vi "Version_Parse.vi"(0 "All_ERD_Data_Bundled_Brass in":T2, 5 "Converted Data Out":T1 {"CRC" format="%04x"; "Length" format="%02x"; "Command" format="%02x"; "Destination" format="%02x"; "Source" format="%02x"}, 11 "Error In":errorcluster) -> (4 "All_ERD_Data_Bundled_Brass out":T2, 15 "Error Out":errorcluster)   [LabVIEW 2019]
uses:
  type defs/All_Bundled_Data_JL.ctl
  type defs/Version.ctl
  type defs/ERD_Always_Show_JL.ctl
  type defs/CSV_File_String_Arrays.ctl
  type defs/Fault Table Array.ctl
  type defs/Fault_Table_Info.ctl
  type defs/Heat Control.ctl
  type defs/ERD_Commercial_Laundry.ctl
  type defs/BootloaderVersion.ctl
  type defs/ERD_RJ45.ctl
  Common/LabVIEW GEA2 Toolkit/GEA3/type defs/Data Out.ctl
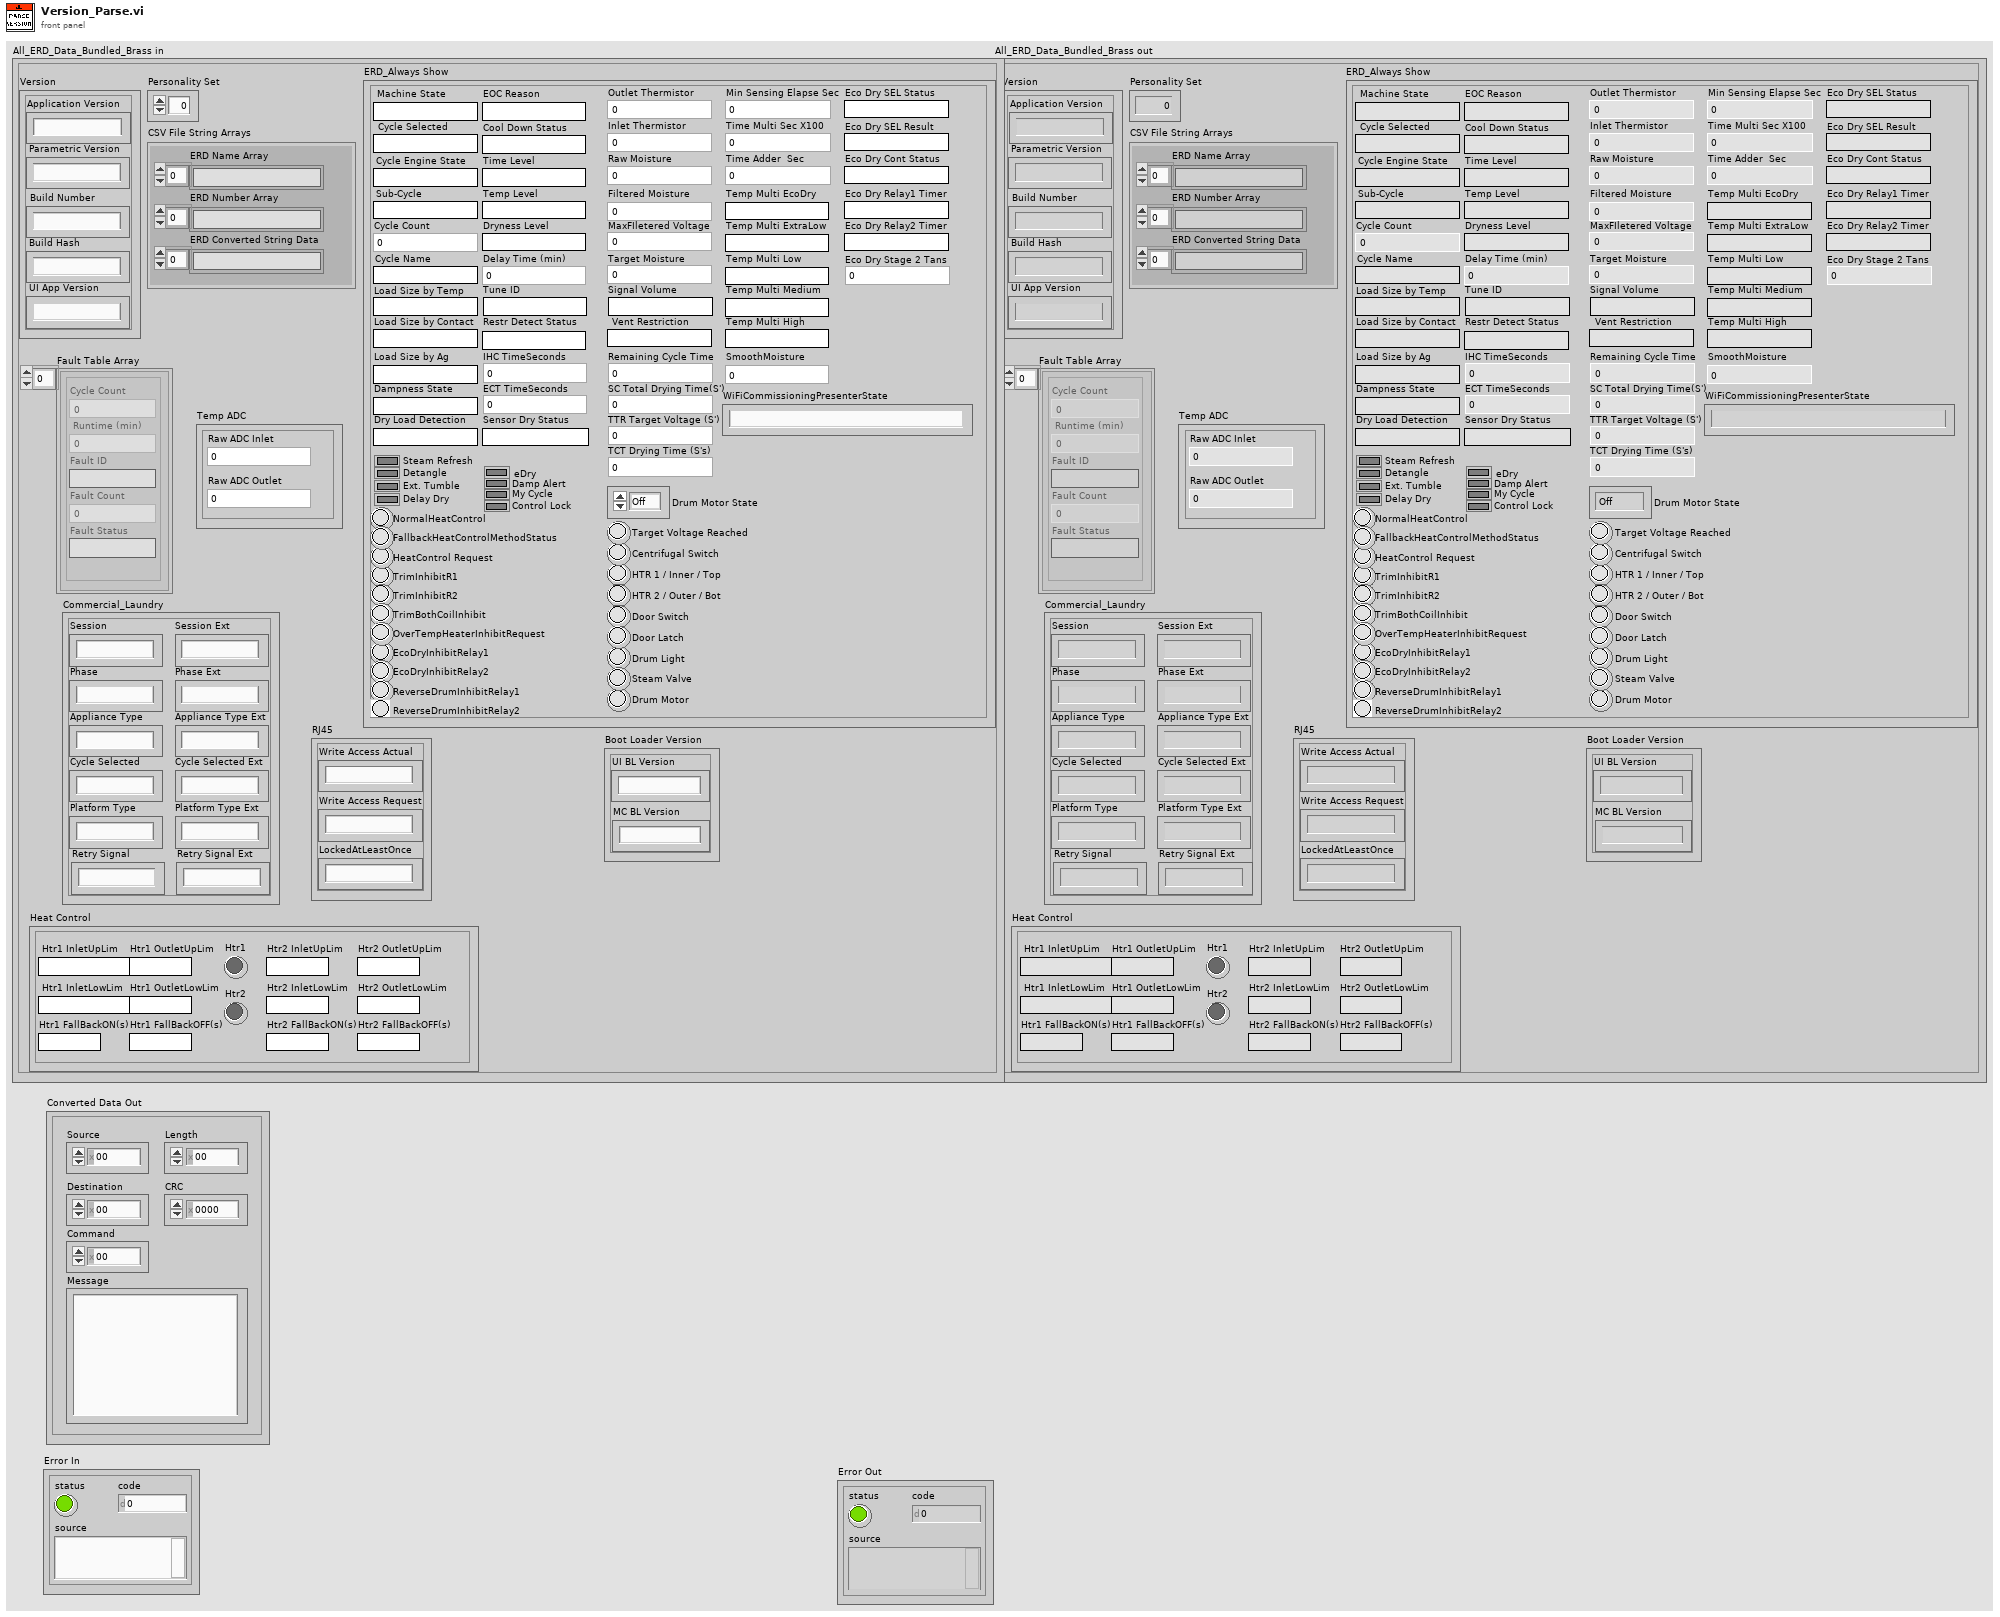
[diagram p1: front panel]
types:
  T1 = typedef "Data Out.ctl" = cluster{"Source":u8, "Destination":u8, "Command":u8, "Length":u8, "CRC":u16, "Message":string}
  T2 = typedef "All_Bundled_Data_JL.ctl" = cluster{"Version":T3, "ERD_Always Show":T4, "Personality Set":u8, "CSV File String Arrays":T5, "Fault Table Array ":T6, "Heat Control":T8, "Temp ADC":cluster{"Raw ADC Outlet":u16, "Raw ADC Inlet":u16}, "Commercial_Laundry":T9, "Boot Loader Version":T10, "RJ45":T11}
  T3 = typedef "Version.ctl" = cluster{"Build Number":string, "Build Hash ":string, "Application Version":string, "Parametric Version":string, "UI App Version":string}
  T4 = typedef "ERD_Always_Show_JL.ctl" = cluster{"Inlet Thermistor":u16, "Machine State":string, "Filtered Moisture":u16, "Cycle Selected":string, "HTR 1 / Inner / Top":bool, "HTR 2 / Outer / Bot":bool, "Door Switch":bool, "Drum Light":bool, "Cycle Engine State":string, "Centrifugal Switch":bool, "Drum Motor":bool, "Cycle Count":u32, "Ext. Tumble":bool, "eDry":bool, "Temp Level":string, "Dryness Level":string, "Time Level":string, "Delay Time (min)":u16, "Steam Refresh":bool, "Damp Alert":bool, "Sub-Cycle":string, "Outlet Thermistor":u16, "Target Moisture":u16, "Remaining Cycle Time":u32, "Raw Moisture":u16, "Cycle Name":string, "My Cycle":bool, "Delay Dry":bool, "Detangle":bool, "Control Lock":bool, "Steam Valve":bool, "Door Latch":bool, "Signal Volume":string, "Tune ID":string, "Restr Detect Status":string, "Vent Restriction":string, "Load Size by Contact":string, "Load Size by Temp":string, "EOC Reason":string, "Sensor Dry Status":string, "Dampness State":string, "Target Voltage Reached":bool, "TrimInhibitR1":bool, "TrimInhibitR2":bool, "TrimBothCoilInhibit":bool, "NormalHeatControl":bool, "HeatControl Request":bool, "Cool Down Status":string, "EcoDryInhibitRelay1":bool, "EcoDryInhibitRelay2":bool, "ReverseDrumInhibitRelay1":bool, "ReverseDrumInhibitRelay2":bool, "OverTempHeaterInhibitRequest":bool, "FallbackHeatControlMethodStatus":bool, "IHC TimeSeconds":u32, "ECT TimeSeconds ":u32, "SC Total Drying Time(S')":u32, "TTR Target Voltage (S')":u32, "TCT Drying Time (S's)":u32, "Drum Motor State":enum16{"Off", "Cw", "Ccw", "Max"}, "Load Size by Ag":string, "MaxFIletered Voltage":u16, "Dry Load Detection":string, "Min Sensing Elapse Sec":u32, "Time Multi Sec X100":u32, "Time Adder  Sec":u32, "Temp Multi EcoDry":string, "Temp Multi ExtraLow":string, "Temp Multi Low ":string, "Temp Multi Medium":string, "Temp Multi High":string, "SmoothMoisture":u16, "Eco Dry SEL Status":string, "Eco Dry SEL Result":string, "Eco Dry Cont Status":string, "Eco Dry Relay1 Timer":string, "Eco Dry Relay2 Timer ":string, "Eco Dry Stage 2 Tans ":u32, "WiFiCommissioningPresenterState":string}
  T5 = typedef "CSV_File_String_Arrays.ctl" = cluster{"ERD Number Array":string[], "ERD Name Array":string[], "ERD Converted String Data":string[]}
  T6 = typedef "Fault Table Array.ctl" = T7[]
  T7 = typedef "Fault_Table_Info.ctl" = cluster{"Cycle Count":u32, " Runtime (min) ":u32, "Fault Status":string, "Fault ID":string, "Fault Count":u16}
  T8 = typedef "Heat Control.ctl" = cluster{"Htr1 InletLowLim":string, "Htr1 InletUpLim":string, "Htr1 OutletLowLim":string, "Htr1 OutletUpLim":string, "Htr1 FallBackON(s)":string, "Htr1 FallBackOFF(s)":string, "Htr1":bool, "Htr2 InletLowLim":string, "Htr2 InletUpLim":string, "Htr2 OutletLowLim":string, "Htr2 OutletUpLim":string, "Htr2 FallBackON(s)":string, "Htr2 FallBackOFF(s)":string, "Htr2":bool}
  T9 = typedef "ERD_Commercial_Laundry.ctl" = cluster{"Session":string, "Phase":string, "Appliance Type":string, "Cycle Selected":string, "Platform Type":string, "Retry Signal":string, "Session Ext":string, "Phase Ext":string, "Appliance Type Ext":string, "Cycle Selected Ext":string, "Platform Type Ext":string, "Retry Signal Ext":string}
  T10 = typedef "BootloaderVersion.ctl" = cluster{"UI BL Version":string, "MC BL Version":string}
  T11 = typedef "ERD_RJ45.ctl" = cluster{"Write Access Actual":string, "Write Access Request":string, "LockedAtLeastOnce":string}
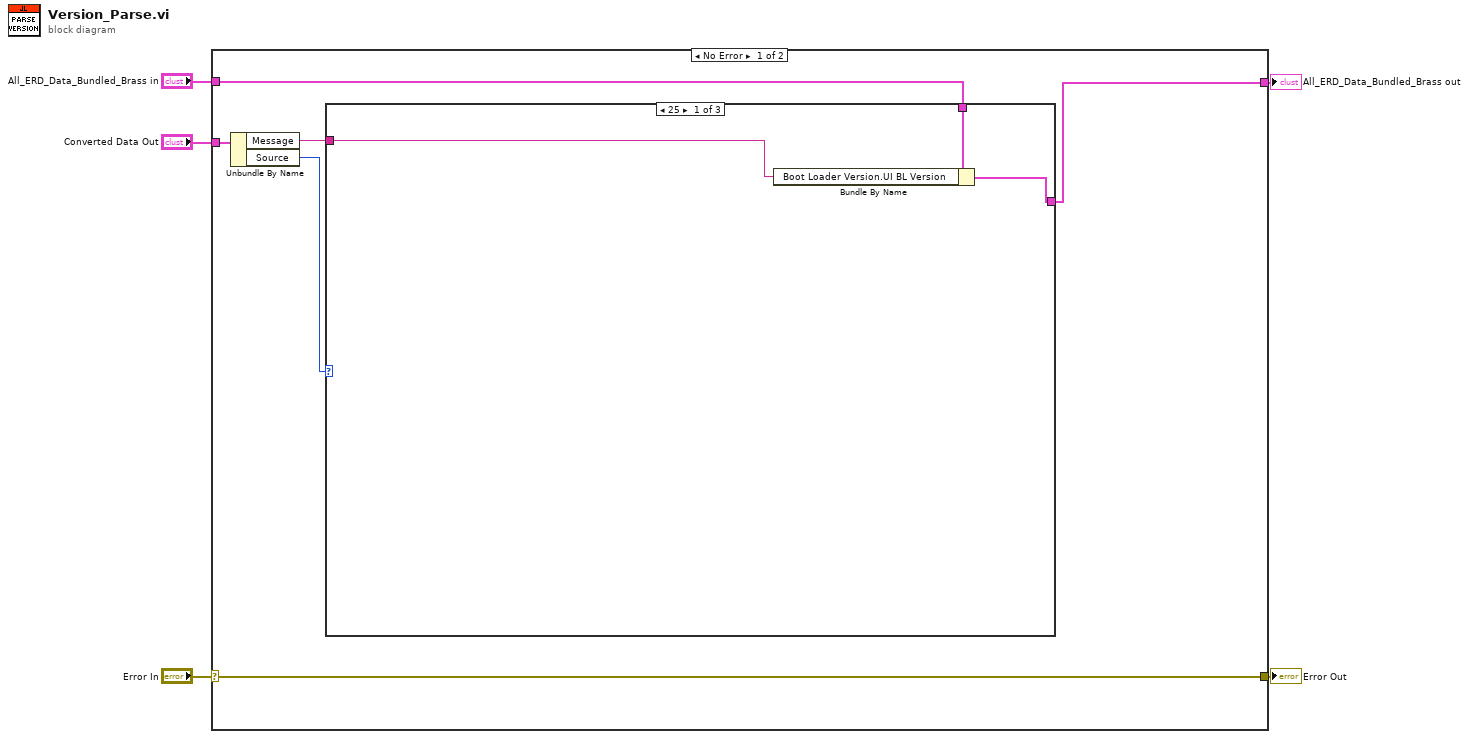
[diagram p0: block diagram]
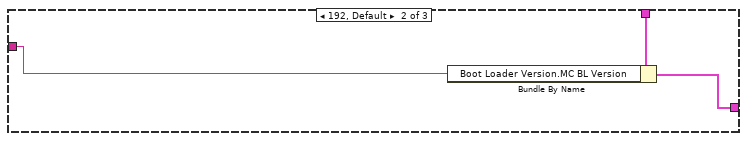
[diagram p2: hidden frame]
diagram:
  n1 = case shown="No Error" "Error In" {
    selector: "Error In" -> [w9 w20]
    tunnel: [w11 w19] -> w5
    tunnel: "All_ERD_Data_Bundled_Brass in" -> [w10 w19]
    tunnel: "Converted Data Out" -> [w8 _]
    tunnel: [w9 w20] -> w1
    frame No Error {
      n2 = Unbundle By Name(w8) -> ("Message"=w7:string, "Source"=w6:u8)
      n3 = case shown="25" w6 {
        tunnel: [w14 w17 w18] -> w11
        tunnel: w10 -> [w13 w16 w18]
        tunnel: w7 -> [w12 w15 _]
        frame 37 {
          n4 = Bundle By Name(cluster=w13, "Boot Loader Version.UI BL Version"=w12) -> (w14:T2)
        }
        frame 192, Default {
          n5 = Bundle By Name(cluster=w16, "Boot Loader Version.MC BL Version"=w15) -> (w17:T2)
        }
        frame 36 {
        }
      }
    }
    frame Error {
    }
  }
  "All_ERD_Data_Bundled_Brass out" <- w5
  "Error Out" <- w1
